vi "iRobot Navigation Target.vi"() -> ()   [LabVIEW 2013]
uses:
  iRobot Sensors.ctl
  iRobot Navigation State Machine.lvsc/StatechartState.ctl
  iRobot Navigation State Machine.lvsc/State.ctl
  <vilib>/userdefined/High Color/IMAQdx.ctl
  iRobot Navigation State Machine.lvsc/Inputs.ctl
  Accelerometer.ctl
  iRobot/Sensor/Sensor Group 6.ctl
  iRobot/Sensor/Bumps + Wheel Drops.ctl
  iRobot/Sensor/Low-Side Driver + Wheel Overcurrent.ctl
  iRobot/Sensor/Buttons.ctl
  iRobot/Sensor/Charging State.ctl
  iRobot/Sensor/Cargo Bay Digital Inputs.ctl
  iRobot/Sensor/Charging Sources Available.ctl
  iRobot/Sensor/OI Mode.ctl
  iRobot Navigation State Machine.lvsc/CompanionDiagram.vi/40/SC Main.vi
  iRobot Navigation State Machine.lvsc/CompanionDiagram.vi/40/Upd State.vi
  iRobot Navigation State Machine.lvsc/CompanionDiagram.vi/40/Trans Graph0.vi
  iRobot Navigation State Machine.lvsc/CompanionDiagram.vi/40/EnterGraphCore.vi
  <vilib>/myRIO/Common/Instrument Driver Framework/myRIO v1.0/UART/vis/myRIO v1.0 Close UART.vi
  iRobot Navigation State Machine.lvsc/CompanionDiagram.vi/40/Trans Graph1.vi
  iRobot Navigation State Machine.lvsc/CompanionDiagram.vi/40/Trans Graph2.vi
  <vilib>/myRIO/Common/Instrument Driver Framework/myRIO v1.0/myRIO v1.1 Open.vi
  iRobot Navigation State Machine.lvsc/CompanionDiagram.vi
  <vilib>/myRIO/Common/Instrument Driver Framework/Utilities/vis/FPGA Ref Manager.vi
  <vilib>/myRIO/Common/Instrument Driver Framework/myRIO v1.0/myRIO v1.0 Reset FPGA.vi
  iRobot Navigation State Machine.lvsc/Trigger.ctl
  <vilib>/Statechart/Infrastructure/RTStatechart/RunTime SCN.xnode
  iRobot Navigation State Machine.lvsc/Outputs.ctl
  iRobot Navigation State Machine.lvsc
  <vilib>/myRIO/Instrument Drivers/Utilities/Utilities.lvlib
  <vilib>/vision/NI_Vision_Development_Module.lvlib
  <vilib>/vision/driver/NI_Vision_Acquisition_Software.lvlib
panel:
  in  "Blue or Luminance":cluster{i32, i32}(slide)={20, 217} scale=0.0..255.0
  in  "Green or Saturation":cluster{i32, i32}(slide)={20, 233} scale=0.0..255.0
  in  "Red 2":cluster{i32, i32}(slide)={42, 99} scale=0.0..255.0
  in  "stop 2":bool
  out "Process Time":dbl
  in  "Green 2":cluster{i32, i32}(slide)={42, 99} scale=0.0..255.0
  in  "Green or Saturation 2":cluster{i32, i32}(slide)={20, 233} scale=0.0..255.0
  in  "Blue or Luminance 2":cluster{i32, i32}(slide)={20, 217} scale=0.0..255.0
  out "Nb Circles Green":i32
  out "Green":bool
  out "Red":bool
  out "Second":T1(plugin-control)
  out "Color Threshold Image":T1(plugin-control)
  out "Remove Obj 2":T1(plugin-control)
  out "Circle":T1(plugin-control)
  out "Nb Circles Red":i32
  out "Cam 2":T1(plugin-control)
  in  "Tab Control":T2(tab)
  out "iRobot Sensors (graphical)":T3 {"Right Wheel (mm/s)" scale=-500.0..500.0; "Left Wheel (mm/s)" scale=-500.0..500.0}
  out "Active States":T5
  out "error out":errorcluster
  in  "Wheel Speed (mm/s)":i16(slide)=100 scale=0.0..500.0
  in  "accel smoothing (0-1)":dbl=0.1
  in  "stop":bool
  out "Target Running":bool
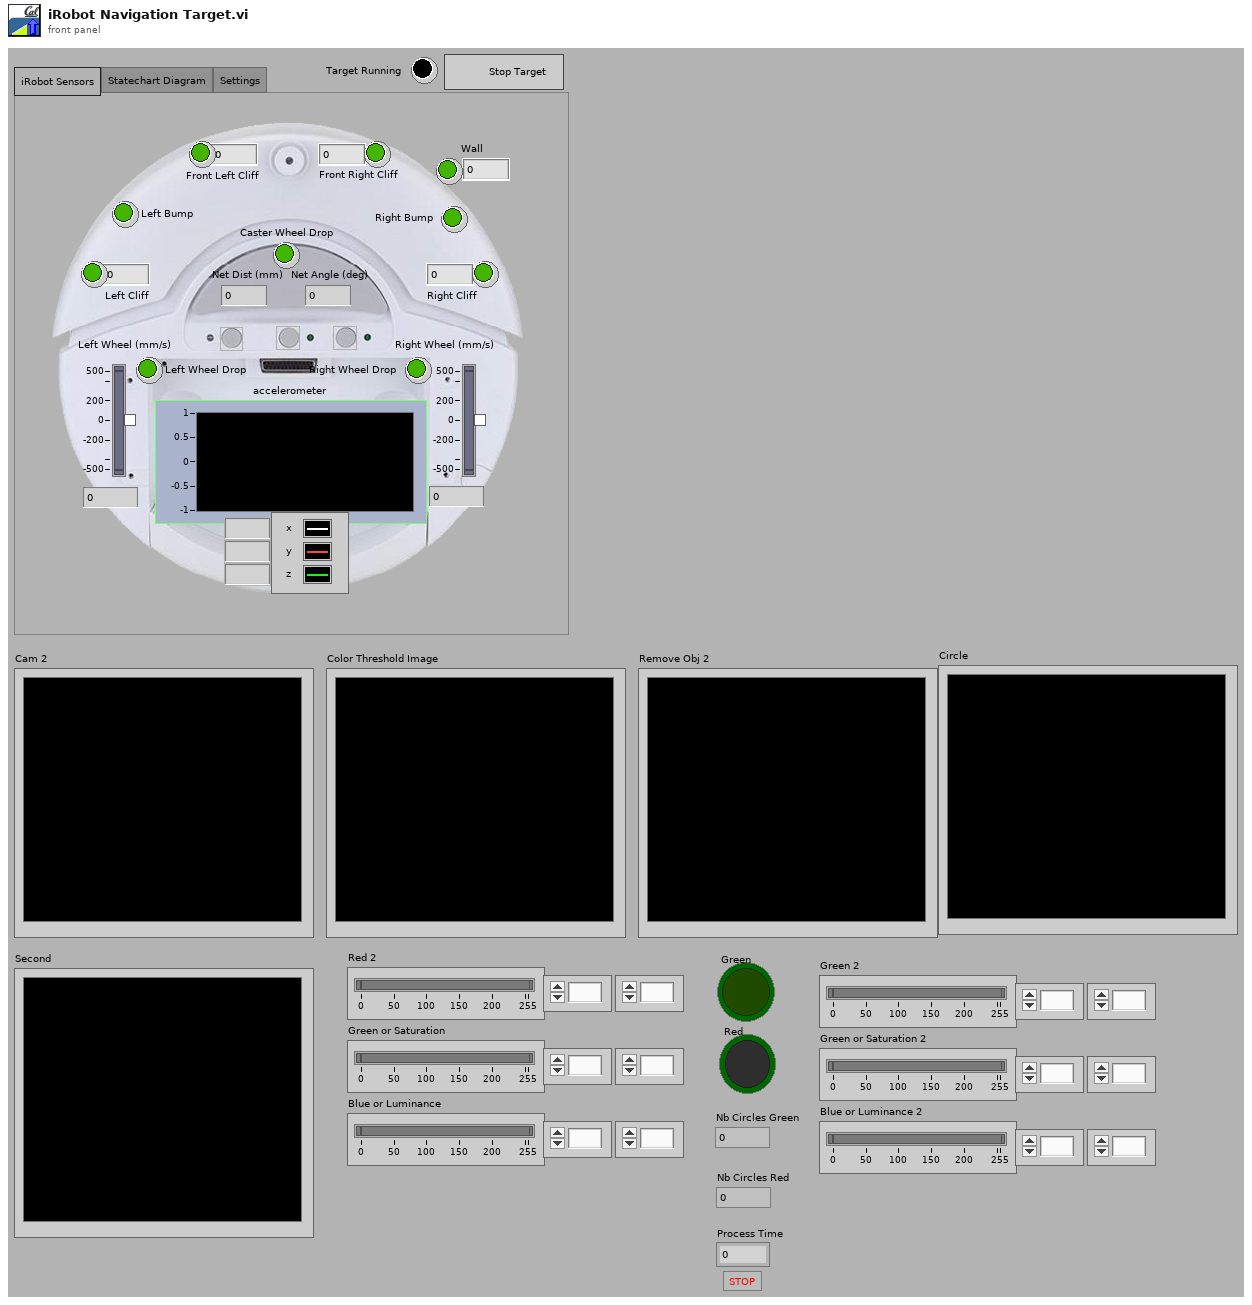
[diagram p1: front panel]
types:
  T1 = typedef "IMAQ Image.ctl" = refnum<image>
  T2 = enum32{"iRobot Sensors", "Statechart Diagram", "Settings"}
  T3 = typedef "iRobot Sensors.ctl" = cluster{"Caster Wheel Drop":bool, "Left Wheel Drop":bool, "Right Wheel Drop":bool, "Left Bump":bool, "Right Bump":bool, "Left Cliff":bool, "Front Left Cliff":bool, "Front Right Cliff":bool, "Right Cliff":bool, "Wall":bool, "Net Dist (mm)":i32, "Net Angle (deg)":i32, "Wall":u16, "Left Cliff":u16, "Front Left Cliff":u16, "Front Right Cliff":u16, "Right Cliff":u16, "Left Wheel (mm/s)":i16, "Right Wheel (mm/s)":i16, "accelerometer":T4}
  T4 = typedef "Accelerometer.ctl" = cluster{"x axis (g)":dbl, "y axis (g)":dbl, "z axis (g)":dbl}
  T5 = typedef "iRobot Navigation State Machine.lvsc/StatechartState.ctl" = T6[]
  T6 = typedef "iRobot Navigation State Machine.lvsc/State.ctl" = enum16{"NI.SC.Initial", "NI.SC.History", "NI.SC.ShallowHistory", "NI.SC.Terminal", "Pause", "Run", "Pause\\Detect Play Button\\Pause;\nWait for\nbutton\nrelease", "Pause\\Detect Play Button\\Unpause;\nwait for\nbutton release", "Pause\\Detect Play Button\\Unpause;\nwait for\nbutton press", "Run\\Detect Obstacles\\Object in front", "Run\\Detect Obstacles\\State", "Run\\Detect Obstacles\\Hit right side", "Run\\Detect Obstacles\\Hit left side", "Run\\Detect Obstacles\\Front Crossing the Line", "Run\\Detect Obstacles\\Right Passing", "Run\\Detect Obstacles\\Left Passing", "Run\\Detect Obstacles\\Hit the line", "Run\\Detect Obstacles\\Drive"}
  T7 = typedef "IMAQdx.ctl" = refnum<k21>
  T8 = typedef "iRobot UART Port Type.ctl" = refnum<visa-resource-name>
  T9 = typedef "iRobot Navigation State Machine.lvsc/Inputs.ctl" = cluster{"net distance (mm)":i32, "net angle (deg)":i32, "Max Wheel Speed (mm/s)":i16, "accelerometer":T4, "iRobot Sensors":T10, "Is Simulator?":bool, "Green":bool, "Red":bool}
  T10 = typedef "Sensor Group 6.ctl" = cluster{"Bumps + Wheel Drops":T11, "Wall":bool, "Cliff Left":bool, "Cliff Front Left":bool, "Cliff Front Right":bool, "Cliff Right":bool, "Virtual Wall":bool, "Low-Side Driver + Wheel Overcurrent":T12, "Infrared":u8, "Buttons":T13, "Distance (mm)":i32, "Angle (deg)":i32, "Charging State":T14, "Voltage (mV)":u16, "Current (mA)":i16, "Battery Temperature (deg C)":i8, "Battery Charge (mAh)":u16, "Battery Capacity (mAh)":u16, "Wall Signal (0-4095)":u16, "Cliff Left Signal (0-4095)":u16, "Cliff Front Left Signal (0-4095)":u16, "Cliff Front Right Signal (0-4095)":u16, "Cliff Right Signal (0-4095)":u16, "Cargo Bay Digital Inputs":T15, "Cargo Bay Analog Signal (0-1023)":u16, "Charging Sources Available":T16, "OI Mode":T17, "Song Number":u8, "Song Playing":bool, "Number of Stream Packets":u8, "Requested Velocity (mm/s)":i16, "Requested Radius (mm)":i16, "Requested Right Wheel Velocity (mm/s)":i16, "Requested Left Wheel Velocity (mm/s)":i16}
  T11 = typedef "Bumps + Wheel Drops.ctl" = cluster{"Wheeldrop Caster":bool, "Wheeldrop Left":bool, "Wheeldrop Right":bool, "Bump Left":bool, "Bump Right":bool}
  T12 = typedef "Low-Side Driver + Wheel Overcurrent.ctl" = cluster{"Low-Side Driver 0":bool, "Low-Side Driver 1":bool, "Low-Side Driver 2":bool, "Left Wheel":bool, "Right Wheel":bool}
  T13 = typedef "Buttons.ctl" = cluster{"Advance":bool, "Play":bool}
  T14 = typedef "Charging State.ctl" = enum16{"Not Charging", "Reconditioning Charging", "Full Charging", "Trickle Charging", "Waiting", "Charging Fault Condition"}
  T15 = typedef "Cargo Bay Digital Inputs.ctl" = cluster{"Digital Input 0":bool, "Digital Input 1":bool, "Digital Input 2":bool, "Digital Input 3":bool, "Device Detect":bool}
  T16 = typedef "Charging Sources Available.ctl" = cluster{"Internal Charger":bool, "Home Base":bool}
  T17 = typedef "OI Mode.ctl" = enum16{"Off", "Passive", "Safe", "Full"}
  T18 = typedef "iRobot Navigation State Machine.lvsc/Outputs.ctl" = cluster{"Left Wheel Speed (mm/s)":i16, "Right Wheel Speed (mm/s)":i16}
  T19 = enum32{"AutoM", "Close", "Dilate", "Erode", "Gradient", "Gradient out", "Gradient in", "Hit miss", "Open", "PClose", "POpen", "Thick", "Thin"}
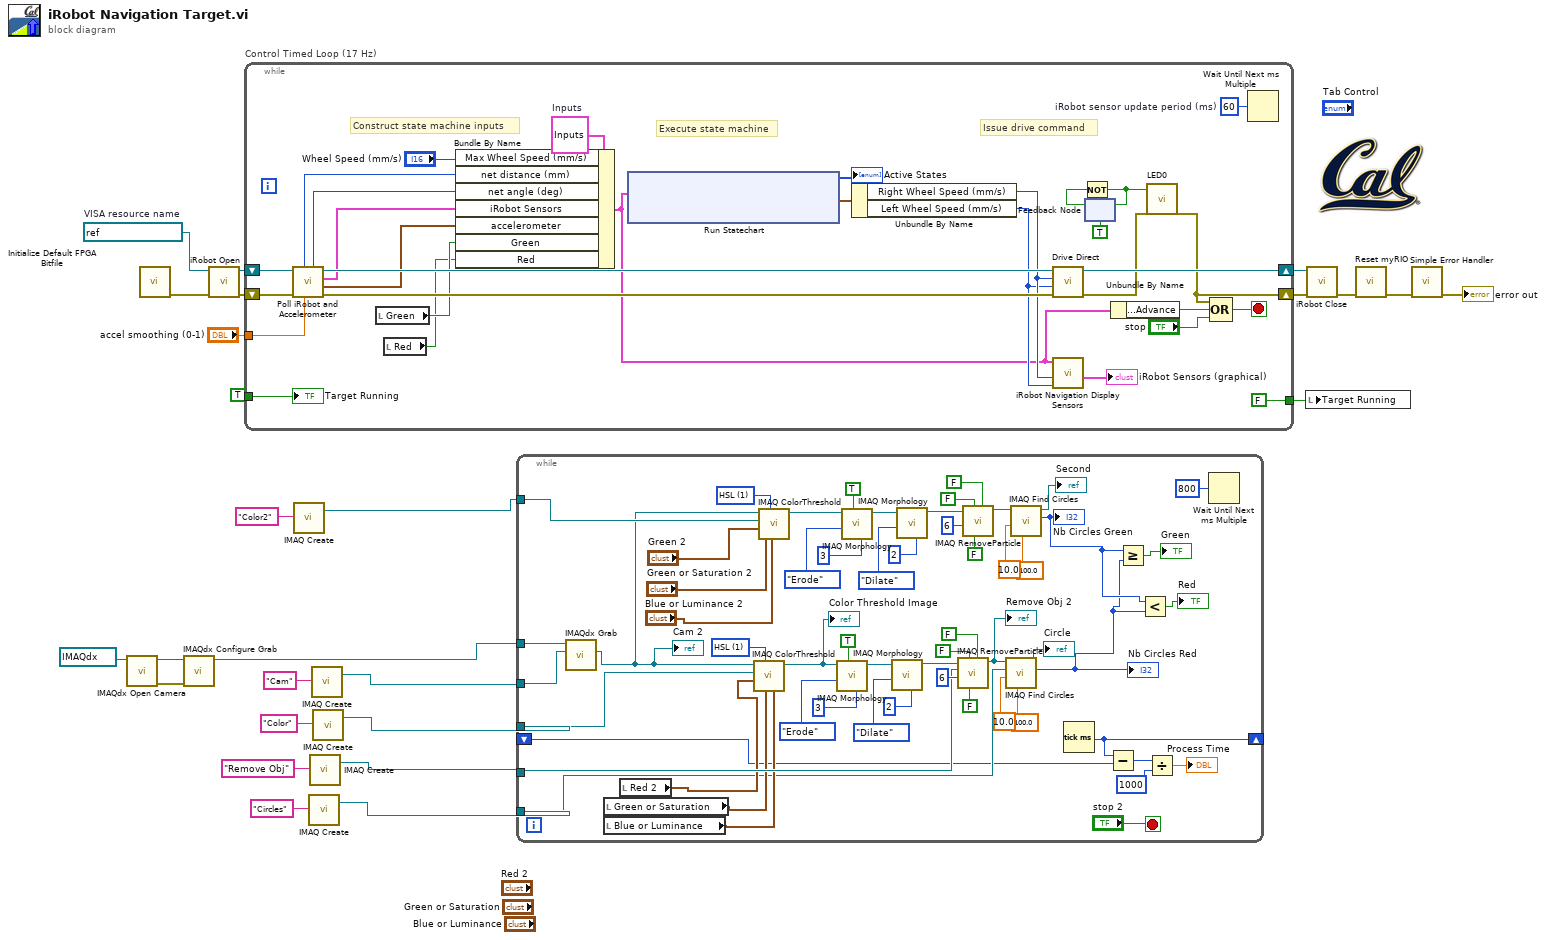
[diagram p0: block diagram]
diagram:
  w20 = refnum<visa-resource-name> "ASRL1::INSTR"  # VISA resource name
  n1 = call <vilib>:"IMAQdx Open Camera.vi"("Session In"=T7 "cam0") -> ("error out"=w9:errorcluster, "Session Out"=w8:T7)  [unwired: 9 in]
  n2 = call <vilib>:"Initialize Default FPGA Bitfile.vi"() -> ("error out"=w18:errorcluster)  [unwired: 11 in]
  n3 = call <vilib>:"IMAQdx Configure Grab.vi"("error in"=w9, "Session In"=w8) -> ("Session Out"=w5:T7)  [unwired: 8 in, 1 out]
  n4 = call "iRobot Open.vi"("error in (no error)"=w18, "UART port in"=w20) -> ("error out"=w25:errorcluster, "UART port out"=w24:T8)  [unwired: 8 in]
  n5 = while "Control Timed Loop (17 Hz)" {
    shift-right: [w57] -> w26
    shift-left: w24 -> [w52]
    shift-right: [w39] -> w21
    shift-left: w25 -> [w51]
    tunnel: TRUE ("stop") -> [w45]
    tunnel: [FALSE ("stop")] -> w22
    tunnel: "accel smoothing (0-1)" -> [w31]
    stop <- w56 stop-if-true
    w29 = u32 60  # iRobot sensor update period (ms)
    w54 = T9 {"net distance (mm)"=0, "net angle (deg)"=0, "Max Wheel Speed (mm/s)"=0, "accelerometer"={"x axis (g)"=0.0, "y axis (g)"=0.0, "z axis (g)"=0.0}, "iRobot Sensors"={"Bumps + Wheel Drops"={"Wheeldrop Caster"=FALSE, "Wheeldrop Left"=FALSE, "Wheeldrop Right"=FALSE, "Bump Left"=FALSE, "Bump Right"=FALSE}, "Wall"=FALSE, "Cliff Left"=FALSE, "Cliff Front Left"=FALSE, "Cliff Front Right"=FALSE, "Cliff Right"=FALSE, "Virtual Wall"=FALSE, "Low-Side Driver + Wheel Overcurrent"={"Low-Side Driver 0"=FALSE, "Low-Side Driver 1"=FALSE, "Low-Side Driver 2"=FALSE, "Left Wheel"=FALSE, "Right Wheel"=FALSE}, "Infrared"=255, "Buttons"={"Advance"=FALSE, "Play"=FALSE}, "Distance (mm)"=0, "Angle (deg)"=0, "Charging State"=enum."Not Charging", "Voltage (mV)"=0, "Current (mA)"=0, "Battery Temperature (deg C)"=0, "Battery Charge (mAh)"=0, "Battery Capacity (mAh)"=0, "Wall Signal (0-4095)"=0, "Cliff Left Signal (0-4095)"=0, "Cliff Front Left Signal (0-4095)"=0, "Cliff Front Right Signal (0-4095)"=0, "Cliff Right Signal (0-4095)"=0, "Cargo Bay Digital Inputs"={"Digital Input 0"=FALSE, "Digital Input 1"=FALSE, "Digital Input 2"=FALSE, "Digital Input 3"=FALSE, "Device Detect"=FALSE}, "Cargo Bay Analog Signal (0-1023)"=0, "Charging Sources Available"={"Internal Charger"=FALSE, "Home Base"=FALSE}, "OI Mode"=enum."Off", "Song Number"=0, "Song Playing"=FALSE, "Number of Stream Packets"=0, "Requested Velocity (mm/s)"=0, "Requested Radius (mm)"=0, "Requested Right Wheel Velocity (mm/s)"=0, "Requested Left Wheel Velocity (mm/s)"=0}, "Is Simulator?"=FALSE, "Green"=FALSE, "Red"=FALSE}  # Inputs
    # "Issue drive command"
    # "Execute state machine"
    # "Construct state machine inputs"
    n6 = call "Poll iRobot and Accelerometer.vi"("accel smoothing (0-1)"=w31, "error in"=w51, "UART port in"=w52) -> ("error out"=w50:errorcluster, "Acceleration (g)"=w30:T4, "iRobot SensorGroup6"=w38:T10, "UART port out"=w49:T8, "net angle (deg)"=w47:i32, "net distance (mm)"=w48:i32)  [unwired: 3 in]
    n7 = local read "Green"() -> (w28:bool)
    n8 = local read "Red"() -> (w27:bool)
    n9 = Bundle By Name(cluster=w54, "Max Wheel Speed (mm/s)"="Wheel Speed (mm/s)", "net distance (mm)"=w48, "net angle (deg)"=w47, "iRobot Sensors"=w38, "accelerometer"=w30, "Green"=w28, "Red"=w27) -> (w33:T9)
    n10 = xnode "Run Statechart"("Inputs"=w33) -> ("Outputs"=w55:T18, "Active States"=→"Active States":T5)  [unwired: 2 in, 1 out]
    n11 = Unbundle By Name(w55) -> ("Right Wheel Speed (mm/s)"=w36:i16, "Left Wheel Speed (mm/s)"=w35:i16)
    n12 = call "Drive Direct.vi"("error in"=w50, "Left Wheel Velocity (mm/s)"=w35, "Right Wheel Velocity (mm/s)"=w36, "UART port in"=w49) -> ("error out"=w40:errorcluster, "UART port out"=w57:T8)  [unwired: 6 in]
    n13 = call "iRobot Navigation Display Sensors.vi"("Left Wheel (mm/s)"=w35, "Right Wheel (mm/s)"=w36, "Statechart Inputs"=w33) -> ("iRobot Sensors (graphical)"=→"iRobot Sensors (graphical)":T3)  [unwired: 6 in]
    n14 = feedback #1(TRUE) -> (w41:bool)
    n15 = Not(x=w41) -> (.not. x?=w42:bool)
    n16 = feedback-in #1(w42) -> ()
    n17 = Unbundle By Name(w33) -> ("iRobot Sensors.Buttons.Advance"=w32:bool)
    n18 = call "LED0"("LED0"=w42, "error in (no error)"=w40) -> ("error out"=w39:errorcluster)  [unwired: 25 in]
    n19 = Compound Arithmetic op=OR(w39, w32, "stop") -> (w56:bool)
    n20 = Wait Until Next ms Multiple(millisecond multiple=w29) -> ()  [unwired: 1 out]
    "Target Running" <- w45
  }
  n21 = call "IMAQ Create"("Image Name"="Color2") -> ("New Image"=w6:T1)  [unwired: 4 in, 1 out]
  n22 = call "IMAQ Create"("Image Name"="Circles") -> ("New Image"=w1:T1)  [unwired: 4 in, 1 out]
  n23 = call "IMAQ Create"("Image Name"="Remove Obj") -> ("New Image"=w2:T1)  [unwired: 4 in, 1 out]
  n24 = call "IMAQ Create"("Image Name"="Cam") -> ("New Image"=w4:T1)  [unwired: 4 in, 1 out]
  n25 = call "IMAQ Create"("Image Name"="Color") -> ("New Image"=w3:T1)  [unwired: 4 in, 1 out]
  n26 = while {
    tunnel: w4 -> [w200]
    tunnel: w3 -> [w199]
    tunnel: w2 -> [w198]
    tunnel: w1 -> [w194]
    shift-right: [w193] -> _
    shift-left: _ -> [w192]
    tunnel: w6 -> [w172]
    tunnel: w5 -> [w163]
    stop <- "stop 2" stop-if-true
    w188 = u16 1 items=["RGB", "HSL", "HSV", "HSI"] ("Color Mode")
    w215 = u16 1 items=["RGB", "HSL", "HSV", "HSI"] ("Color Mode")
    n27 = call <vilib>:"IMAQdx Grab.vi"("Image In"=w200, "Session In"=w163) -> ("Image Out"=w164:T1)  [unwired: 6 in, 3 out]
    "Cam 2" <- w164
    n28 = local read "Green or Saturation"() -> (w196:cluster{i32, i32})
    n29 = local read "Blue or Luminance"() -> (w197:cluster{i32, i32})
    n30 = local read "Red 2"() -> (w195:cluster{i32, i32})
    n31 = call "IMAQ ColorThreshold"("Blue or Luma or Val or Inten Range"=w197, "Green or Sat Range"=w196, "Color Mode"=w215, "Red or Hue Range"=w195, "Image Dst"=w199, "Image Src"=w164) -> ("Image Dst Out"=w167:T1)  [unwired: 4 in, 1 out]
    "Color Threshold Image" <- w167
    n32 = call "IMAQ ColorThreshold"("Blue or Luma or Val or Inten Range"="Blue or Luminance 2", "Green or Sat Range"="Green or Saturation 2", "Color Mode"=w188, "Red or Hue Range"="Green 2", "Image Dst"=w172, "Image Src"=w164) -> ("Image Dst Out"=w174:T1)  [unwired: 4 in, 1 out]
    n33 = call "IMAQ Morphology"("Number of iterations (1)"=3, "Square/Hexa (Square)"=TRUE, "Operation"=T19."Erode", "Image Src"=w167) -> ("Image Dst Out"=w211:T1)  [unwired: 6 in, 1 out]
    n34 = call "IMAQ Morphology"("Number of iterations (1)"=3, "Square/Hexa (Square)"=TRUE, "Operation"=T19."Erode", "Image Src"=w174) -> ("Image Dst Out"=w184:T1)  [unwired: 6 in, 1 out]
    n35 = call "IMAQ Morphology"("Number of iterations (1)"=2, "Operation"=T19."Dilate", "Image Src"=w211) -> ("Image Dst Out"=w208:T1)  [unwired: 7 in, 1 out]
    n36 = call "IMAQ Morphology"("Number of iterations (1)"=2, "Operation"=T19."Dilate", "Image Src"=w184) -> ("Image Dst Out"=w181:T1)  [unwired: 7 in, 1 out]
    n37 = call "IMAQ RemoveParticle"("Connectivity 4/8 (8)"=FALSE, "Low Pass/High Pass (Low)"=FALSE, "Square/Hexa (Square)"=FALSE, "Number of Erosion"=6, "Image Dst"=w198, "Image Src"=w208) -> ("Image Dst Out"=w166:T1)  [unwired: 4 in, 1 out]
    "Remove Obj 2" <- w166
    n38 = call "IMAQ RemoveParticle"("Connectivity 4/8 (8)"=FALSE, "Low Pass/High Pass (Low)"=FALSE, "Square/Hexa (Square)"=FALSE, "Number of Erosion"=6, "Image Src"=w181) -> ("Image Dst Out"=w173:T1)  [unwired: 5 in, 1 out]
    n39 = call "IMAQ Find Circles"("Max Radius"=sgl 100.0, "Min Radius"=sgl 10.0, "Image Dst"=w194, "Image Src"=w166) -> ("Nb Circles"=w158:i32, "Image Dst Out"=→"Circle":T1)  [unwired: 4 in, 2 out]
    "Nb Circles Red" <- w158
    n40 = call "IMAQ Find Circles"("Max Radius"=sgl 100.0, "Min Radius"=sgl 10.0, "Image Src"=w173) -> ("Nb Circles"=w159:i32, "Image Dst Out"=→"Second":T1)  [unwired: 5 in, 2 out]
    "Nb Circles Green" <- w159
    n41 = Tick Count (ms)() -> (millisecond timer value=w193:u32)
    n42 = Subtract(x=w193, y=w192) -> (x-y=w191:u32)
    n43 = Greater Or Equal?(x=w159, y=w158) -> (x >= y?=→"Green":bool)
    n44 = Less?(x=w159, y=w158) -> (x < y?=→"Red":bool)
    n45 = Divide(x=w191, y=u32 1000) -> (x/y=→"Process Time":dbl)
    n46 = Wait Until Next ms Multiple(millisecond multiple=u32 800) -> ()  [unwired: 1 out]
  }
  n47 = local write "Target Running"(w22) -> ()
  n48 = call "iRobot Close.vi"("error in"=w21, "UART port in"=w26) -> ("error out"=w15:errorcluster)  [unwired: 9 in]
  n49 = call <vilib>:"Reset myRIO.vi"("error in (no error)"=w15) -> ("error out"=w19:errorcluster)  [unwired: 10 in]
  n50 = call <vilib>:"Simple Error Handler.vi"("error in (no error)"=w19) -> ("error out"=→"error out":errorcluster)  [unwired: 4 in, 4 out]
